vi "TestingEnvironment.vi"() -> ()   [LabVIEW 2023]
panel:
  out "String":string
  in  "2":bool
  out "Array":dbl[](array[numeric])
  in  "1":bool
  in  "16":bool
  in  "15":bool
  in  "13":bool
  in  "14":bool
  in  "12":bool
  in  "11":bool
  in  "10":bool
  in  "9":bool
  in  "8":bool
  in  "7":bool
  in  "6":bool
  in  "5":bool
  in  "4":bool
  in  "3":bool
  in  "1":bool
  in  "2":bool
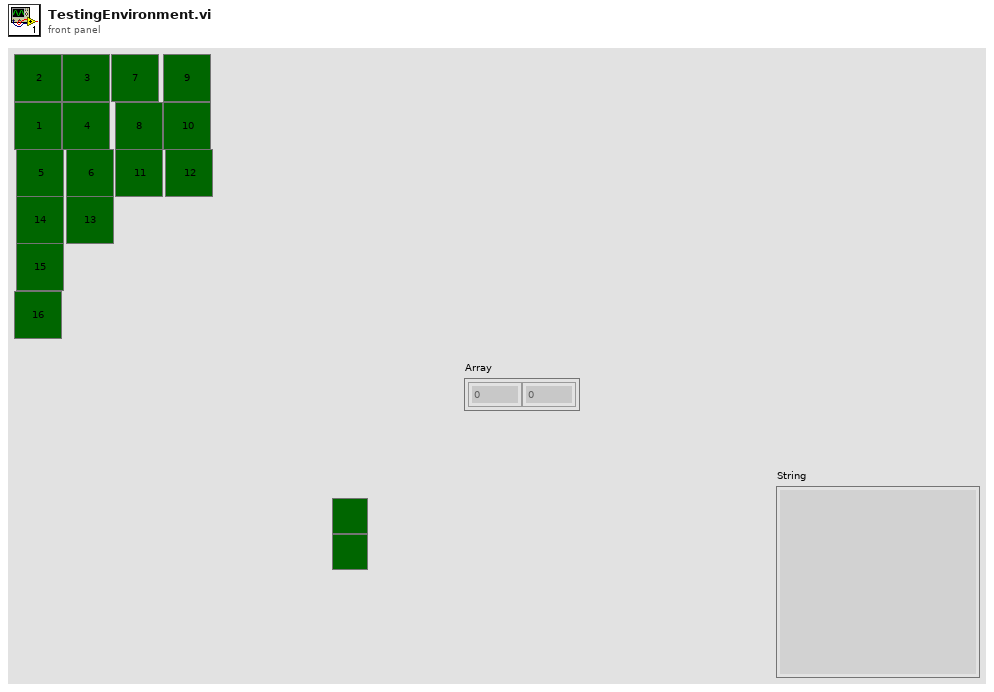
[diagram p1: front panel]
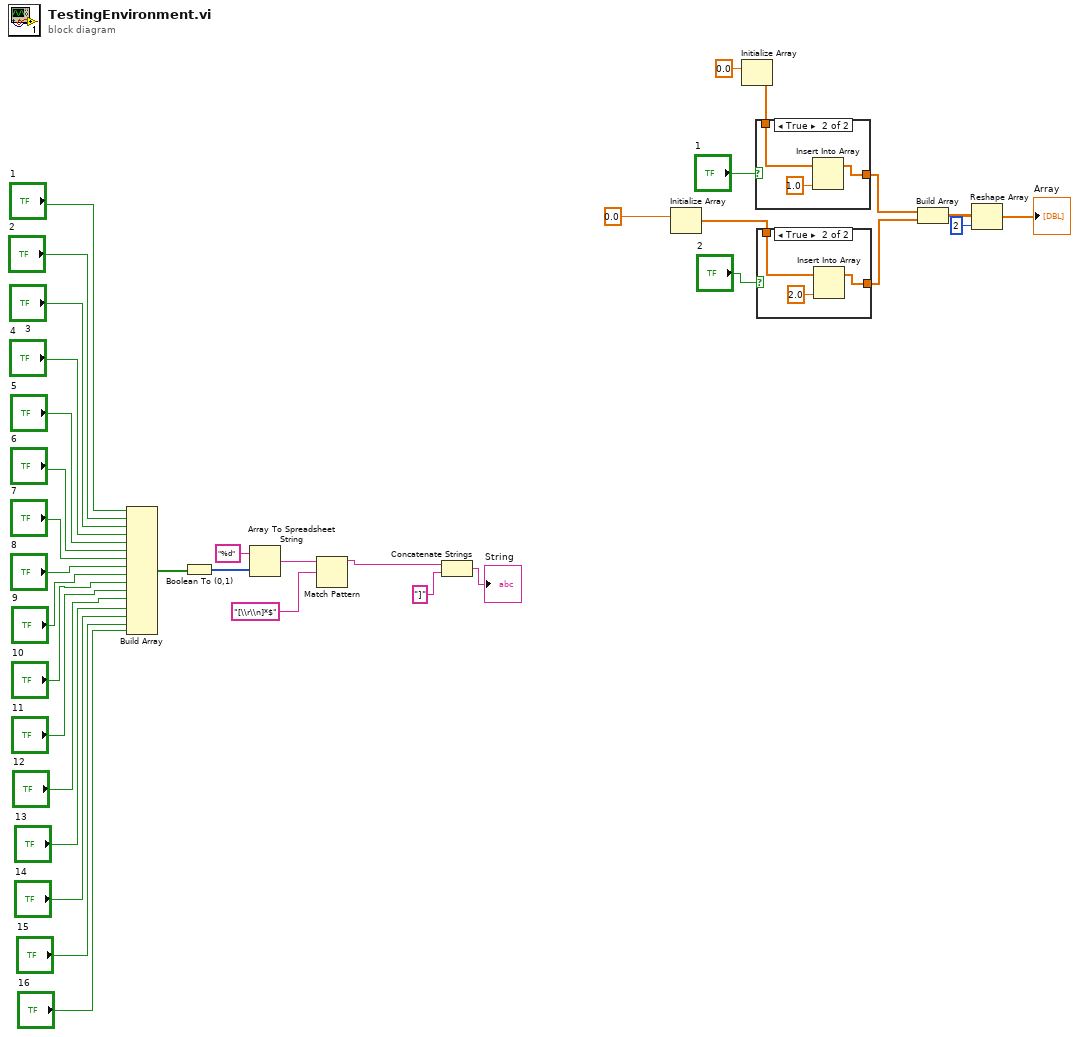
[diagram p0: block diagram]
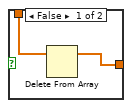
[diagram p2: hidden frame]
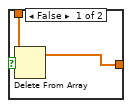
[diagram p3: hidden frame]
diagram:
  n1 = Build Array("1", "2", "3", "4", "5", "6", "7", "8", "9", "10", "11", "12", "13", "14", "15", "16") -> (w19:bool[])
  n2 = Boolean To (0,1)(Boolean=w19) -> (0, 1=w7:i16[])
  n3 = Array To Spreadsheet String(array=w7, 3:"%d" ("format string")) -> (spreadsheet string=w3:string)  [unwired: 1 in]
  n4 = Match Pattern(string=w3, regular expression="[\\r\\n]*$") -> (before substring=w1:string)  [unwired: 1 in, 3 out]
  n5 = Concatenate Strings(w1, "]" ("string")) -> (→"String":string)
  n6 = Initialize Array(0.0 ("element")) -> (w11:dbl[])  [unwired: 1 in]
  n7 = Initialize Array(0.0 ("element")) -> (w15:dbl[])  [unwired: 1 in]
  n8 = case shown="True" "1" {
    tunnel: w15 -> [w37 w40]
    tunnel: [w36 w39] -> w14
    frame False {
      n9 = Delete From Array(array=w37) -> (array with subset deleted=w36:dbl[])  [unwired: 2 in, 1 out]
    }
    frame True {
      n10 = Insert Into Array(array=w40, new element=1.0 ("new element/subarray")) -> (w39:dbl[])  [unwired: 1 in]
    }
  }
  n11 = case shown="True" "2" {
    tunnel: w11 -> [w42 w45]
    tunnel: [w41 w44] -> w13
    frame False {
      n12 = Delete From Array(array=w42) -> (array with subset deleted=w41:dbl[])  [unwired: 2 in, 1 out]
    }
    frame True {
      n13 = Insert Into Array(array=w45, new element=2.0 ("new element/subarray")) -> (w44:dbl[])  [unwired: 1 in]
    }
  }
  n14 = Build Array(w14, w13) -> (w10:dbl[][])
  n15 = Reshape Array(w10, 2 ("dimension size")) -> (→"Array":dbl[])
